vi "PLC.Dial800.Read Config.vi"(8 "error in (no error)":errorcluster, 11 "Config Folder":path=path "C:/MTE/Circle Test/Config") -> (0 "error out":errorcluster, 2 "OPC Server":T1={"IP"="localhost", "Topic"="Stn800", "Server"="RSLinx OPC Server", "VarRoot"="Program:Stn001_90_OffloadMain", "TestPCArray"="TestPC", "VarNames"={"SN"="SN", "Reset"="Reset", "HeartbeatPLC"="HeartbeatPLC", "HeartbeatPC"="HeartbeatTestPC", "Start"="Start", "Running"="Running", "Done"="Done", "Pass"="Pass"}}, 3 "Nest":i32)   [LabVIEW 2018]
uses:
  PLC.Dial800.OPC Server Config.ctl
  PLC.Dial800.VarNames.ctl
  Utils/Errors/Error.Error Code List.ctl
  <vilib>/Utility/config.llb/Read Key (I32).vi
  <vilib>/Utility/config.llb/Read Key (String).vi
  <vilib>/Utility/config.llb/NI_LVConfig.lvlib
  <vilib>/KATE/Files/File Utils.lvlib
panel:
  # "(Access path)"
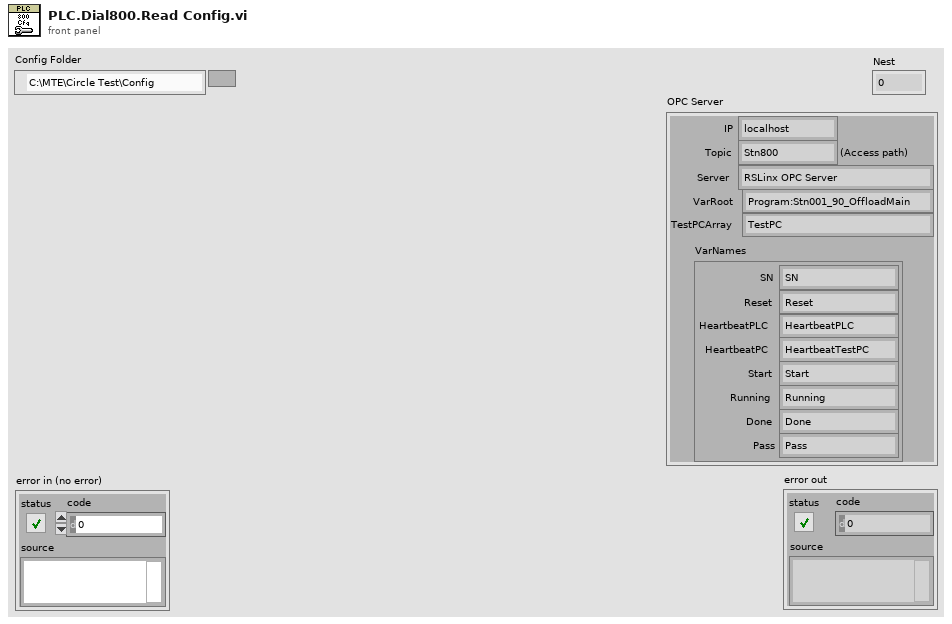
[diagram p1: front panel]
types:
  T1 = typedef "PLC.Dial800.OPC Server Config.ctl" = cluster{"IP":string, "Topic":string, "Server":string, "VarRoot":string, "TestPCArray":string, "VarNames":T2}
  T2 = typedef "PLC.Dial800.VarNames.ctl" = cluster{"SN":string, "Reset":string, "HeartbeatPLC":string, "HeartbeatPC":string, "Start":string, "Running":string, "Done":string, "Pass":string}
  T3 = typedef "Error.Error Code List.ctl" = i32
  T4 = typedef "NI_LVConfig.lvlib/Config Data RefNum.ctl" = refnum<k1>
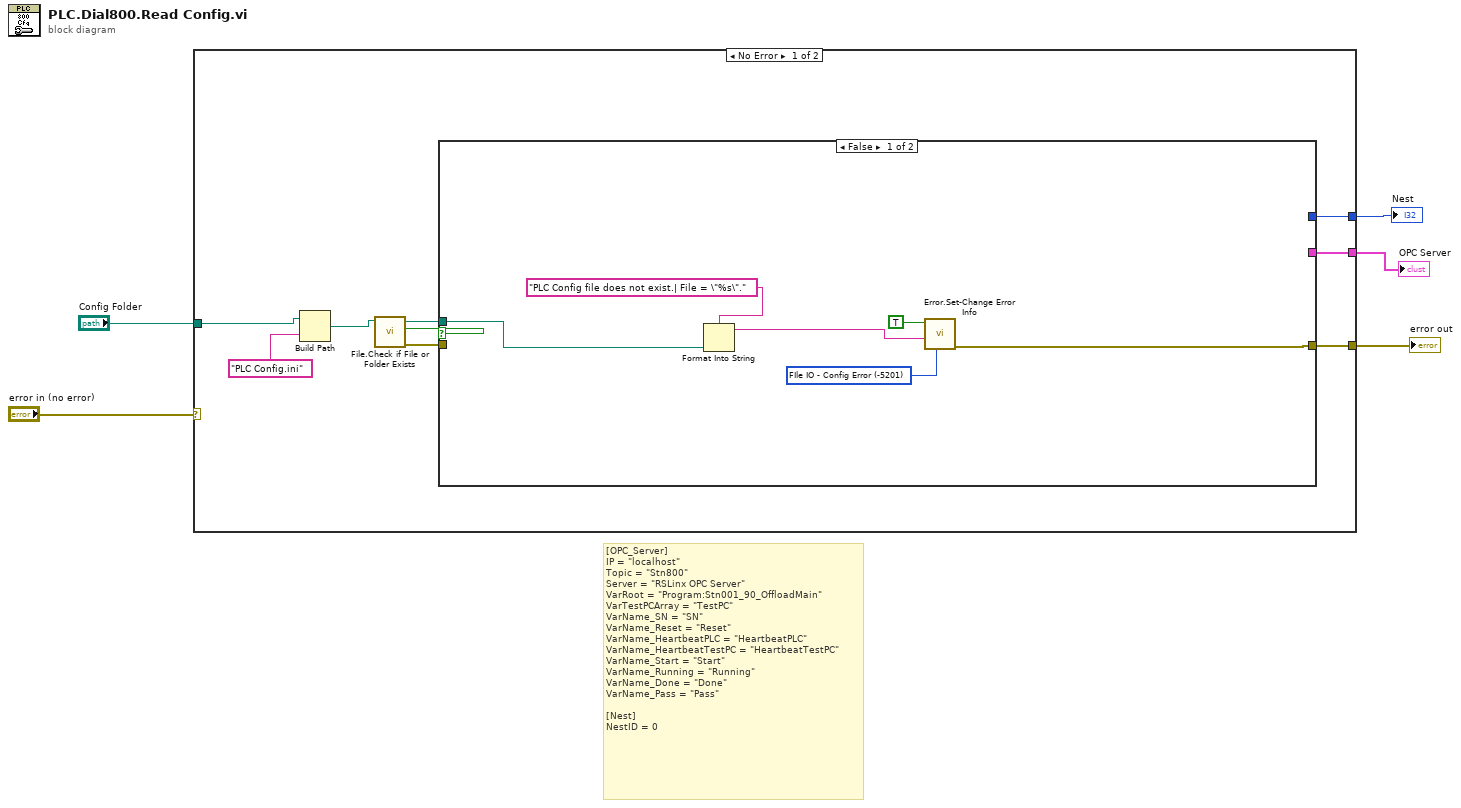
[diagram p0: block diagram]
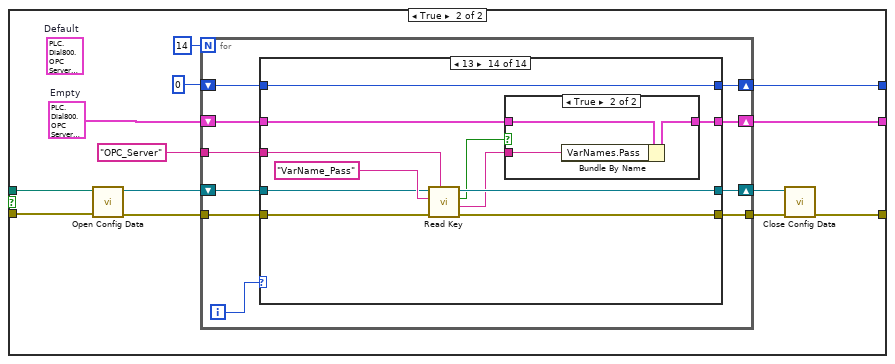
[diagram p2: hidden frame]
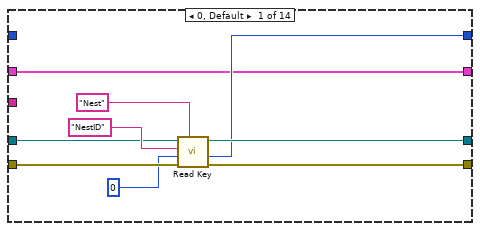
[diagram p3: hidden frame]
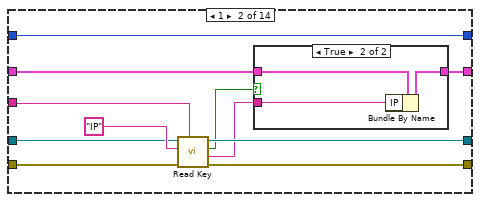
[diagram p4: hidden frame]
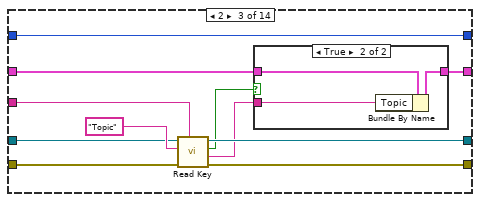
[diagram p6: hidden frame]
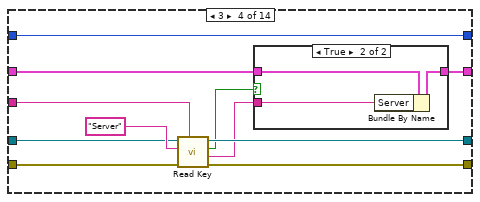
[diagram p8: hidden frame]
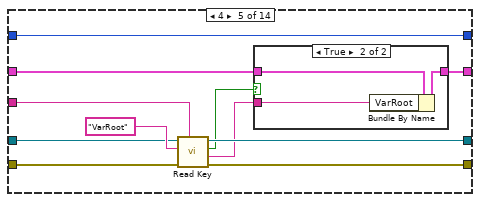
[diagram p10: hidden frame]
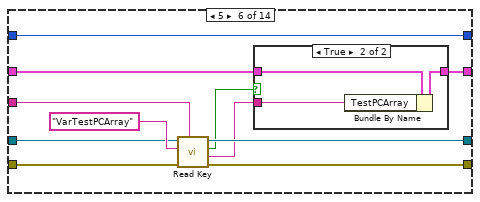
[diagram p12: hidden frame]
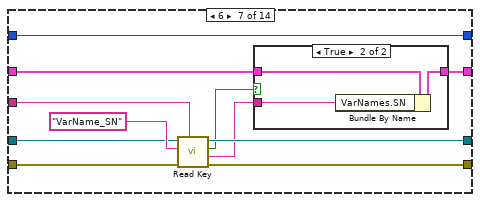
[diagram p14: hidden frame]
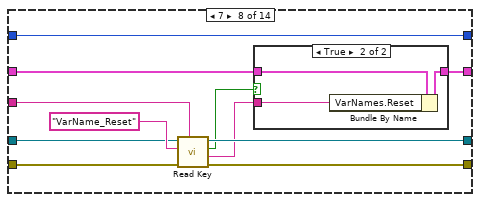
[diagram p16: hidden frame]
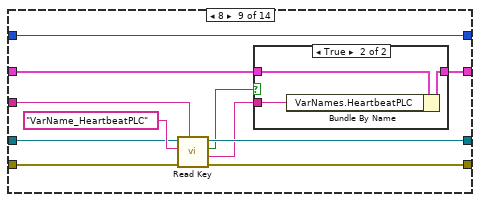
[diagram p18: hidden frame]
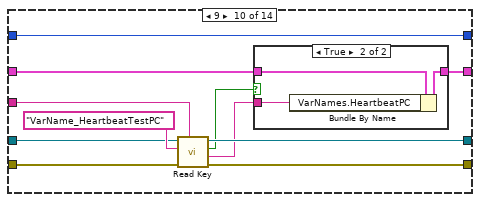
[diagram p20: hidden frame]
diagram:
  # "[OPC_Server]\nIP = \"localhost\"\nTopic = \"Stn800\"\nServer = \"RSLinx OPC Server\"\nVarRoot = \"Program:Stn001_90_OffloadMain\"\nVarTestPCArray = \"TestPC\"\nVarName_SN = \"SN\"\nVarName_Reset = \"Reset\"\nVarName_HeartbeatPLC = \"HeartbeatPLC\"\nVarName_HeartbeatTestPC = \"HeartbeatTestPC\"\nVarName_Start = \"Start\"\nVarName_Running = \"Running\"\nVarName_Done = \"Done\"\nVarName_Pass = \"Pass\"\n\n[Nest]\nNestID = 0"
  n1 = case shown="No Error" "error in (no error)" {
    selector: "error in (no error)" -> [_ w248]
    tunnel: [w14 w248] -> w4
    tunnel: "Config Folder" -> [w13 _]
    tunnel: [w7 _] -> w2
    tunnel: [w6 _] -> w1
    frame No Error {
      n2 = Build Path(base path=w13, name or relative path="PLC Config.ini") -> (appended path=w11:path)
      n3 = call <vilib>:"File.Check if File or Folder Exists.vi"("Path"=w11) -> ("error out"=w8:errorcluster, "Exists"=w9:bool, "Dup Path"=w10:path)  [unwired: 6 in, 2 out]
      n4 = case shown="False" w9 {
        tunnel: [w20 w33] -> w14
        tunnel: w10 -> [w15 w32]
        tunnel: w8 -> [_ w28]
        tunnel: [_ w25] -> w7
        tunnel: [_ w24] -> w6
        frame False {
          w19 = T3 -5201 items=["No Error"=0, "Abort"=-2, "Misc"=-5000, "Fixture Error"=-5100, "File IO - General"=-5200, "FIle IO - Config Error"=-5201, "Instrument - General"=-5300, "Instrument - Serial Com"=-5301, "Instrument - Camera"=-5302, "Instrument - PS"=-5303, "Instrument - Oscilloscope"=-5304, "Instrument - Function Gen"=-5305, "Instrument - Load"=-5306, "Instrument - Meter"=-5307, "Instrument - Power Control"=-5308, "Instrument - Motion"=-5309, "Instrument - RF"=-5310, "System Exe"=-5400, "Image Processing"=-5500, "Communication"=-5600, "Script - Syntax Error"=-6000, "Script - Invalid Name or Param"=-6100, "Script - Timeout"=-6200, "Invalid Data"=-6300] ("Std Code")
          n5 = Format Into String(format string="PLC Config file does not exist.| File = \"%s\"." ("Description"), w15) -> (resulting string=w16:string)  [unwired: 2 in, 1 out]
          n6 = call "Error.Set-Change Error Info.vi"("Std Code"=w19, "Description"=w16, "Set Error"=TRUE) -> ("error out"=w20:errorcluster)  [unwired: 8 in]
        }
        frame True {
          (unwired) T1 {"IP"="localhost", "Topic"="Stn800", "Server"="RSLinx OPC Server", "VarRoot"="Program:Stn001_90_OffloadMain", "TestPCArray"="TestPC", "VarNames"={"SN"="SN", "Reset"="Reset", "HeartbeatPLC"="HeartbeatPLC", "HeartbeatPC"="HeartbeatTestPC", "Start"="Start", "Running"="Running", "Done"="Done", "Pass"="Pass"}}  # Default
          w26 = T1 {"IP"="", "Topic"="", "Server"=" ", "VarRoot"="", "TestPCArray"="", "VarNames"={"SN"="", "Reset"="", "HeartbeatPLC"="", "HeartbeatPC"="", "Start"="", "Running"="", "Done"="", "Pass"=""}}  # Empty
          n7 = call <vilib>:"Open Config Data.vi"("error in (no error)"=w28, "configuration file path"=w32) -> ("error out"=w27:errorcluster, "refnum"=w29:T4)  [unwired: 7 in, 1 out]
          n8 = for {
            N: 14 -> [_]
            tunnel: [w43] -> w31
            shift-right: [w42] -> w30
            shift-left: w29 -> [w41]
            tunnel: w27 -> [w40]
            shift-right: [w35] -> w25
            shift-left: w26 -> [w37]
            shift-right: [w39] -> w24
            shift-left: 0 -> [w36]
            tunnel: "OPC_Server" -> [w34]
            i -> [w38]
            n9 = case shown="13" w38 {
              tunnel: [w52 w63 w78 w93 w108 w123 w138 w153 w168 w183 w198 w213 w228 w243] -> w43
              tunnel: [w51 w62 w77 w92 w107 w122 w137 w152 w167 w182 w197 w212 w227 w242] -> w42
              tunnel: w41 -> [w48 w60 w75 w90 w105 w120 w135 w150 w165 w180 w195 w210 w225 w240]
              tunnel: w40 -> [w47 w59 w74 w89 w104 w119 w134 w149 w164 w179 w194 w209 w224 w239]
              tunnel: [w45 w58 w73 w88 w103 w118 w133 w148 w163 w178 w193 w208 w223 w238] -> w39
              tunnel: w37 -> [w44 w57 w72 w87 w102 w117 w132 w147 w162 w177 w192 w207 w222 w237]
              tunnel: w36 -> [_ w58 w73 w88 w103 w118 w133 w148 w163 w178 w193 w208 w223 w238]
              tunnel: [w44 w56 w71 w86 w101 w116 w131 w146 w161 w176 w191 w206 w221 w236] -> w35
              tunnel: w34 -> [_ w53 w68 w83 w98 w113 w128 w143 w158 w173 w188 w203 w218 w233]
              frame 0, Default {
                n10 = call-poly <vilib>:"Read Key.vi"("section"="Nest", "error in (no error)"=w47, "default value"=0, "key"="NestID", "refnum"=w48) -> ("error out"=w52:errorcluster, "value"=w45:i32, "refnum out"=w51:T4)  [unwired: 3 in, 1 out]
              }
              frame 1 {
                n11 = call-poly <vilib>:"Read Key.vi"("section"=w53, "error in (no error)"=w59, "key"="IP", "refnum"=w60) -> ("error out"=w63:errorcluster, "value"=w55:string, "found?"=w54:bool, "refnum out"=w62:T4)  [unwired: 4 in]
                n12 = case shown="True" w54 {
                  tunnel: w57 -> [w64 w67]
                  tunnel: [w64 w66] -> w56
                  tunnel: w55 -> [_ w65]
                  frame False {
                  }
                  frame True {
                    n13 = Bundle By Name(cluster=w67, "IP"=w65) -> (w66:T1)
                  }
                }
              }
              frame 2 {
                n14 = call-poly <vilib>:"Read Key.vi"("section"=w68, "error in (no error)"=w74, "key"="Topic", "refnum"=w75) -> ("error out"=w78:errorcluster, "value"=w70:string, "found?"=w69:bool, "refnum out"=w77:T4)  [unwired: 4 in]
                n15 = case shown="True" w69 {
                  tunnel: w72 -> [w79 w82]
                  tunnel: [w79 w81] -> w71
                  tunnel: w70 -> [_ w80]
                  frame False {
                  }
                  frame True {
                    n16 = Bundle By Name(cluster=w82, "Topic"=w80) -> (w81:T1)
                  }
                }
              }
              frame 3 {
                n17 = call-poly <vilib>:"Read Key.vi"("section"=w83, "error in (no error)"=w89, "key"="Server", "refnum"=w90) -> ("error out"=w93:errorcluster, "value"=w85:string, "found?"=w84:bool, "refnum out"=w92:T4)  [unwired: 4 in]
                n18 = case shown="True" w84 {
                  tunnel: w87 -> [w94 w97]
                  tunnel: [w94 w96] -> w86
                  tunnel: w85 -> [_ w95]
                  frame False {
                  }
                  frame True {
                    n19 = Bundle By Name(cluster=w97, "Server"=w95) -> (w96:T1)
                  }
                }
              }
              frame 4 {
                n20 = call-poly <vilib>:"Read Key.vi"("section"=w98, "error in (no error)"=w104, "key"="VarRoot", "refnum"=w105) -> ("error out"=w108:errorcluster, "value"=w100:string, "found?"=w99:bool, "refnum out"=w107:T4)  [unwired: 4 in]
                n21 = case shown="True" w99 {
                  tunnel: w102 -> [w109 w112]
                  tunnel: [w109 w111] -> w101
                  tunnel: w100 -> [_ w110]
                  frame False {
                  }
                  frame True {
                    n22 = Bundle By Name(cluster=w112, "VarRoot"=w110) -> (w111:T1)
                  }
                }
              }
              frame 5 {
                n23 = call-poly <vilib>:"Read Key.vi"("section"=w113, "error in (no error)"=w119, "key"="VarTestPCArray", "refnum"=w120) -> ("error out"=w123:errorcluster, "value"=w115:string, "found?"=w114:bool, "refnum out"=w122:T4)  [unwired: 4 in]
                n24 = case shown="True" w114 {
                  tunnel: w117 -> [w124 w127]
                  tunnel: [w124 w126] -> w116
                  tunnel: w115 -> [_ w125]
                  frame False {
                  }
                  frame True {
                    n25 = Bundle By Name(cluster=w127, "TestPCArray"=w125) -> (w126:T1)
                  }
                }
              }
              frame 6 {
                n26 = call-poly <vilib>:"Read Key.vi"("section"=w128, "error in (no error)"=w134, "key"="VarName_SN", "refnum"=w135) -> ("error out"=w138:errorcluster, "value"=w130:string, "found?"=w129:bool, "refnum out"=w137:T4)  [unwired: 4 in]
                n27 = case shown="True" w129 {
                  tunnel: w132 -> [w139 w142]
                  tunnel: [w139 w141] -> w131
                  tunnel: w130 -> [_ w140]
                  frame False {
                  }
                  frame True {
                    n28 = Bundle By Name(cluster=w142, "VarNames.SN"=w140) -> (w141:T1)
                  }
                }
              }
              frame 7 {
                n29 = call-poly <vilib>:"Read Key.vi"("section"=w143, "error in (no error)"=w149, "key"="VarName_Reset", "refnum"=w150) -> ("error out"=w153:errorcluster, "value"=w145:string, "found?"=w144:bool, "refnum out"=w152:T4)  [unwired: 4 in]
                n30 = case shown="True" w144 {
                  tunnel: w147 -> [w154 w157]
                  tunnel: [w154 w156] -> w146
                  tunnel: w145 -> [_ w155]
                  frame False {
                  }
                  frame True {
                    n31 = Bundle By Name(cluster=w157, "VarNames.Reset"=w155) -> (w156:T1)
                  }
                }
              }
              frame 8 {
                n32 = call-poly <vilib>:"Read Key.vi"("section"=w158, "error in (no error)"=w164, "key"="VarName_HeartbeatPLC", "refnum"=w165) -> ("error out"=w168:errorcluster, "value"=w160:string, "found?"=w159:bool, "refnum out"=w167:T4)  [unwired: 4 in]
                n33 = case shown="True" w159 {
                  tunnel: w162 -> [w169 w172]
                  tunnel: [w169 w171] -> w161
                  tunnel: w160 -> [_ w170]
                  frame False {
                  }
                  frame True {
                    n34 = Bundle By Name(cluster=w172, "VarNames.HeartbeatPLC"=w170) -> (w171:T1)
                  }
                }
              }
              frame 9 {
                n35 = call-poly <vilib>:"Read Key.vi"("section"=w173, "error in (no error)"=w179, "key"="VarName_HeartbeatTestPC", "refnum"=w180) -> ("error out"=w183:errorcluster, "value"=w175:string, "found?"=w174:bool, "refnum out"=w182:T4)  [unwired: 4 in]
                n36 = case shown="True" w174 {
                  tunnel: w177 -> [w184 w187]
                  tunnel: [w184 w186] -> w176
                  tunnel: w175 -> [_ w185]
                  frame False {
                  }
                  frame True {
                    n37 = Bundle By Name(cluster=w187, "VarNames.HeartbeatPC"=w185) -> (w186:T1)
                  }
                }
              }
              frame 10 {
                n38 = call-poly <vilib>:"Read Key.vi"("section"=w188, "error in (no error)"=w194, "key"="VarName_Start", "refnum"=w195) -> ("error out"=w198:errorcluster, "value"=w190:string, "found?"=w189:bool, "refnum out"=w197:T4)  [unwired: 4 in]
                n39 = case shown="True" w189 {
                  tunnel: w192 -> [w199 w202]
                  tunnel: [w199 w201] -> w191
                  tunnel: w190 -> [_ w200]
                  frame False {
                  }
                  frame True {
                    n40 = Bundle By Name(cluster=w202, "VarNames.Start"=w200) -> (w201:T1)
                  }
                }
              }
              frame 11 {
                n41 = call-poly <vilib>:"Read Key.vi"("section"=w203, "error in (no error)"=w209, "key"="VarName_Running", "refnum"=w210) -> ("error out"=w213:errorcluster, "value"=w205:string, "found?"=w204:bool, "refnum out"=w212:T4)  [unwired: 4 in]
                n42 = case shown="True" w204 {
                  tunnel: w207 -> [w214 w217]
                  tunnel: [w214 w216] -> w206
                  tunnel: w205 -> [_ w215]
                  frame False {
                  }
                  frame True {
                    n43 = Bundle By Name(cluster=w217, "VarNames.Running"=w215) -> (w216:T1)
                  }
                }
              }
              frame 12 {
                n44 = call-poly <vilib>:"Read Key.vi"("section"=w218, "error in (no error)"=w224, "key"="VarName_Done", "refnum"=w225) -> ("error out"=w228:errorcluster, "value"=w220:string, "found?"=w219:bool, "refnum out"=w227:T4)  [unwired: 4 in]
                n45 = case shown="True" w219 {
                  tunnel: w222 -> [w229 w232]
                  tunnel: [w229 w231] -> w221
                  tunnel: w220 -> [_ w230]
                  frame False {
                  }
                  frame True {
                    n46 = Bundle By Name(cluster=w232, "VarNames.Done"=w230) -> (w231:T1)
                  }
                }
              }
              frame 13 {
                n47 = call-poly <vilib>:"Read Key.vi"("section"=w233, "error in (no error)"=w239, "key"="VarName_Pass", "refnum"=w240) -> ("error out"=w243:errorcluster, "value"=w235:string, "found?"=w234:bool, "refnum out"=w242:T4)  [unwired: 4 in]
                n48 = case shown="True" w234 {
                  tunnel: w237 -> [w244 w247]
                  tunnel: [w244 w246] -> w236
                  tunnel: w235 -> [_ w245]
                  frame False {
                  }
                  frame True {
                    n49 = Bundle By Name(cluster=w247, "VarNames.Pass"=w245) -> (w246:T1)
                  }
                }
              }
            }
          }
          n50 = call <vilib>:"Close Config Data.vi"("error in (no error)"=w31, "refnum"=w30) -> ("error out"=w33:errorcluster)  [unwired: 8 in, 1 out]
        }
      }
    }
    frame Error {
    }
  }
  "error out" <- w4
  "OPC Server" <- w2
  "Nest" <- w1
